vi "Read Password.vi"(4 "Error In":errorcluster, 7 "Config Data In":refnum<class "Config Data.lvclass">) -> (0 "Error Out":errorcluster, 2 "Password":string, 3 "Config Data Out":refnum<class "Config Data.lvclass">)   [LabVIEW 2014, in "Config Data.lvlib" / "Config Data.lvclass"]
uses:
  Config Data.lvclass
  Config Data.lvclass/Config Data.ctl
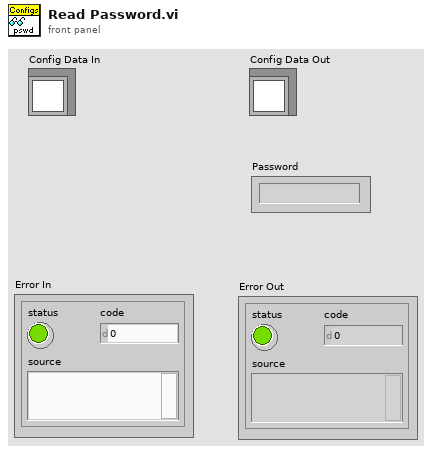
[diagram p1: front panel]
types:
  T1 = typedef "Config Data.lvlib/Config Data.lvclass/Config Mgr Data.ctl" = cluster{"User ID":string, "Password":string}
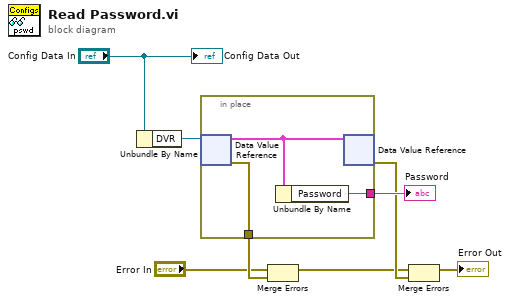
[diagram p0: block diagram]
diagram:
  n1 = Unbundle By Name("Config Data In") -> ("DVR"=w7:refnum<data-value>)
  n2 = in-place {
    in-place-border: [w11] -> w6
    in-place-border: [w9] -> w5
    n3 = in-place-dvr #1(w7) -> (w10:T1, w9:errorcluster)
    n4 = Unbundle By Name(w10) -> ("Password"=w11:string)
    n5 = in-place-dvr #1(w10) -> (w3:errorcluster)  [unwired: 1 out]
  }
  "Password" <- w6
  n6 = Merge Errors("Error In", w5) -> (w2:errorcluster)
  n7 = Merge Errors(w2, w3) -> (→"Error Out":errorcluster)
  "Config Data Out" <- "Config Data In"
